vi "JSON Unflatten.vi"(7 "Variant Type":variant, 8 "error in (no error)":errorcluster, 10 "Root Path ([]=Root)":string[](array[string]), 11 "JSON in":string) -> (0 "error out":errorcluster, 1 "Exists?":bool, 3 "Variant out":variant)   [LabVIEW 2019, in "labview_json.lvlib"]
doc: "Imports a <b>JSON</b> string to a <b>Variant</b>. If <b>Variant Type</b> is not specified, this returns the native JSON data types. Specify the <b>Root Path</b> to get a nested object key or array index.\nCreated by: Ryan Pacini"
uses:
  labview_json.lvlib
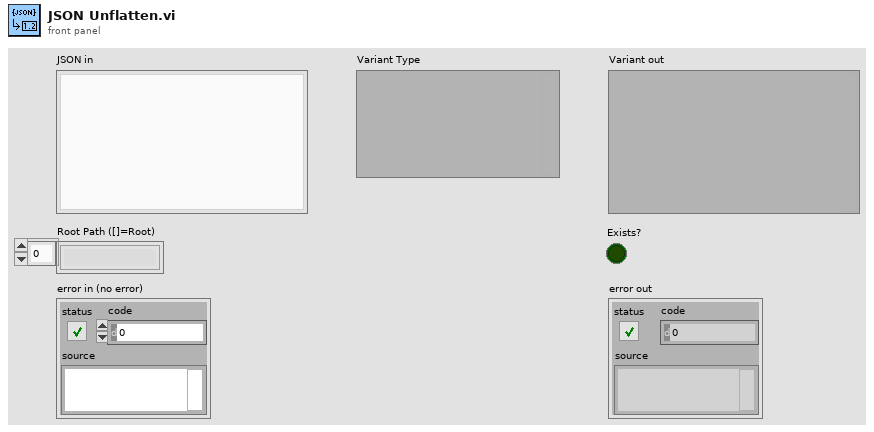
[diagram p1: front panel]
types:
  T1 = typedef "labview_json.lvlib/Element.ctl" = cluster{"Key":string, "Type":T2, "Value":variant}
  T2 = typedef "labview_json.lvlib/Element Type.ctl" = enum8{"NULL", "BOOL", "INT", "UINT", "FLOAT", "STRING", "ARRAY", "OBJECT", "SKIP"}
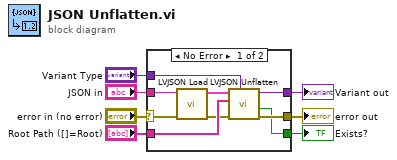
[diagram p0: block diagram]
diagram:
  n1 = case shown="No Error" "error in (no error)" {
    selector: "error in (no error)" -> [w16 w18]
    tunnel: [w10 w18] -> w6
    tunnel: "JSON in" -> [w15 _]
    tunnel: [w9 w17] -> w4
    tunnel: "Variant Type" -> [w11 w17]
    tunnel: "Root Path ([]=Root)" -> [w14 _]
    tunnel: [w8 _] -> w1
    frame No Error {
      n2 = call "LVJSON Load.vi"("error in (no error)"=w16, "JSON in"=w15) -> ("error out"=w13:errorcluster, "Root Element out"=w12:T1)  [unwired: 7 in, 1 out]
      n3 = call "LVJSON Unflatten.vi"("Variant Type"=w11, "error in (no error)"=w13, "Root Path ([]=Root)"=w14, "Root Element in"=w12) -> ("error out"=w10:errorcluster, "Exists?"=w8:bool, "Variant out"=w9:variant)  [unwired: 4 in, 1 out]
    }
    frame Error {
    }
  }
  "error out" <- w6
  "Variant out" <- w4
  "Exists?" <- w1
